vi "Append_Suffiix.vi"(1 "Results file":path) -> (0 "appended path":path)   [LabVIEW 2010]
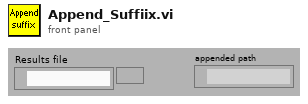
[diagram p1: front panel]
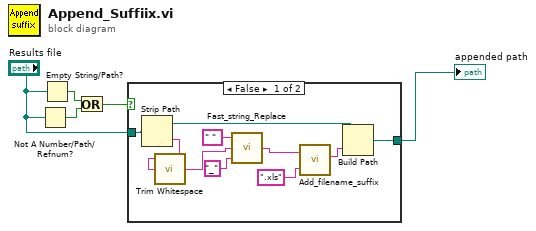
[diagram p0: block diagram]
diagram:
  n1 = Not A Number/Path/Refnum?(number/path/refnum="Results file") -> (NaN/Path/Refnum?=w3:bool)
  n2 = Empty String/Path?(string/path="Results file") -> (empty?=w2:bool)
  n3 = Or(x=w2, y=w3) -> (x .or. y?=w1:bool)
  n4 = case shown="False" w1 {
    tunnel: [w12 w16] -> w5
    tunnel: "Results file" -> [w8 w16]
    frame False {
      n5 = Strip Path(path=w8) -> (stripped path=w9:path, name=w7:string)
      n6 = call <vilib>:"Trim Whitespace.vi"("string"=w7) -> ("trimmed string"=w6:string)  [unwired: 1 in]
      n7 = call "Fast_string_Replace.vi"("Replace match with:"="_", "Input String"=w6, "regular expression"=" ") -> ("Output String"=w15:string)  [unwired: 2 out]
      n8 = call "Add_filename_suffix.vi"("Filename"=w15, "Suffix to add"=".xls") -> ("Filename out"=w10:string)  [unwired: 3 out]
      n9 = Build Path(base path=w9, name or relative path=w10) -> (appended path=w12:path)
    }
    frame True {
    }
  }
  "appended path" <- w5
